vi "FL_Get_Run_Length.vi"(2 "Run Lengths bin array":dbl[](array[numeric]), 3 "Speed lower threshold, mm/s":dbl=8.0 format="%#_13g", 4 "Run Lengts distribution array in":u32[](array[numeric]), 5 "Speed, mm/s":dbl format="%#_13g") -> (0 "Run Lengts distribution array out":u32[](array[numeric]), 1 "Run Length, m":dbl)   [LabVIEW 2016]
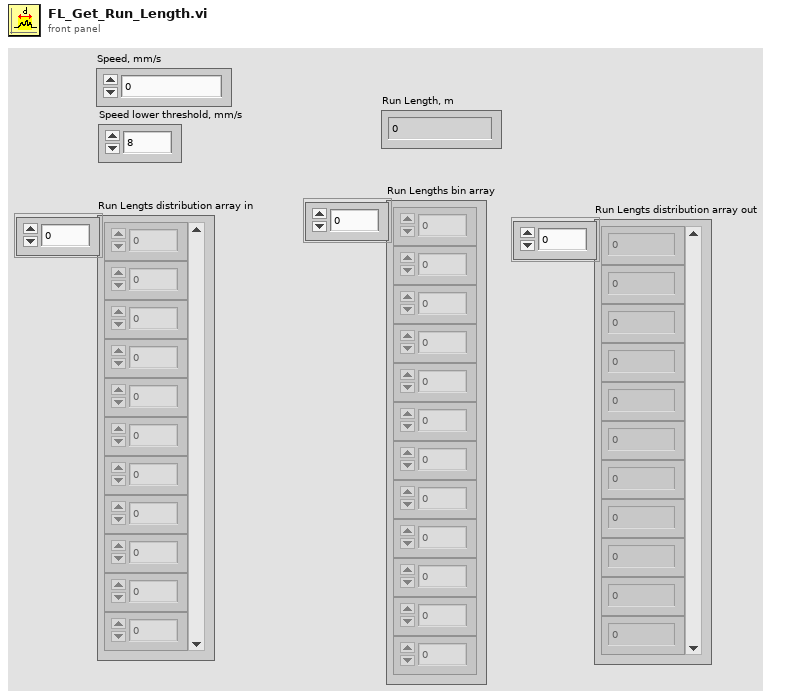
[diagram p1: front panel]
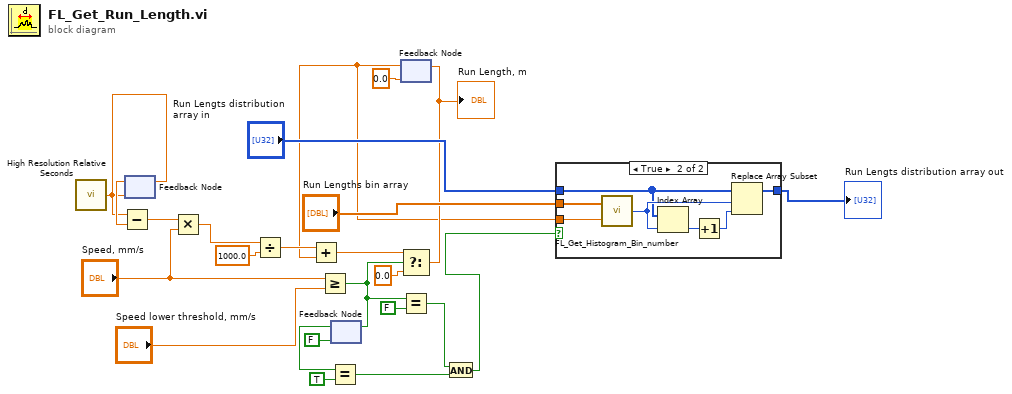
[diagram p0: block diagram]
diagram:
  n1 = call <vilib>:"High Resolution Relative Seconds.vi"() -> ("relative seconds"=w16:dbl)
  n2 = feedback #1(w16) -> (w20:dbl)
  n3 = Subtract(x=w16, y=w20) -> (x-y=w22:dbl)
  n4 = feedback-in #1(w16) -> ()
  n5 = Multiply(x=w22, y="Speed, mm/s") -> (x*y=w24:dbl)
  n6 = Divide(x=w24, y=1000.0) -> (x/y=w15:dbl)
  n7 = Greater Or Equal?(x="Speed, mm/s", y="Speed lower threshold, mm/s") -> (x >= y?=w12:bool)
  n8 = feedback-in #2(w12) -> ()
  n9 = feedback #2(FALSE) -> (w10:bool)
  n10 = Equal?(x=w10, y=TRUE) -> (x = y?=w7:bool)
  n11 = feedback #3(0.0) -> (w1:dbl)
  n12 = Add(x=w15, y=w1) -> (x+y=w18:dbl)
  n13 = Select(t=w18, s=w12, f=0.0) -> (s? t:f=w4:dbl)
  "Run Length, m" <- w4
  n14 = feedback-in #3(w4) -> ()
  n15 = Equal?(x=w12, y=FALSE) -> (x = y?=w8:bool)
  n16 = And(x=w8, y=w7) -> (x .and. y?=w2:bool)
  n17 = case shown="True" w2 {
    tunnel: "Run Lengts distribution array in" -> [w25 w29]
    tunnel: "Run Lengths bin array" -> [_ w28]
    tunnel: w1 -> [_ w27]
    tunnel: [w25 w26] -> w3
    frame False {
    }
    frame True {
      n18 = call "FL_Get_Histogram_Bin_number.vi"("Current value"=w27, "Bins array"=w28) -> ("Bin assignment"=w31:i32)
      n19 = Index Array(array=w29, index=w31) -> (element=w32:u32)
      n20 = Increment(x=w32) -> (x+1=w30:u32)
      n21 = Replace Array Subset(array=w29, new element=w30, index=w31) -> (w26:u32[])
    }
  }
  "Run Lengts distribution array out" <- w3
